vi "difference.vi"(8 "prePicMemory":refnum<k21>, 9 "curPixel":fxp<+,8,8>, 10 "addressInMemory":u16) -> (3 "data Out":fxp<+/-,9,9>)   [LabVIEW 2016]
uses:
  <vilib>/rvi/FXPMathLib/FxpSub/XNode/nifxpmath_Sub.xnode
  <vilib>/rvi/FXPMathLib/sim/FxpSim.dll
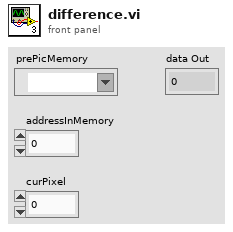
[diagram p1: front panel]
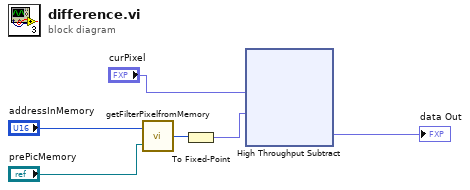
[diagram p0: block diagram]
diagram:
  n1 = call "getFilterPixelfromMemory.vi"("Memory in"="prePicMemory", "addressInMemory"="addressInMemory") -> ("Data Out"=w2:u8)
  n2 = To Fixed-Point(number=w2) -> (fixed-point=w1:fxp<+,8,8>)  [unwired: 1 in]
  n3 = xnode "High Throughput Subtract"("x"="curPixel", "y"=w1) -> ("x-y"=→"data Out":fxp<+/-,9,9>)
